vi "SeCrTs-RD AI Indexing.vi"(11 "AI Config":T1) -> ()   [LabVIEW 2022 SP3]
panel:
  out "Ai Index Element":i32[](array[numeric])
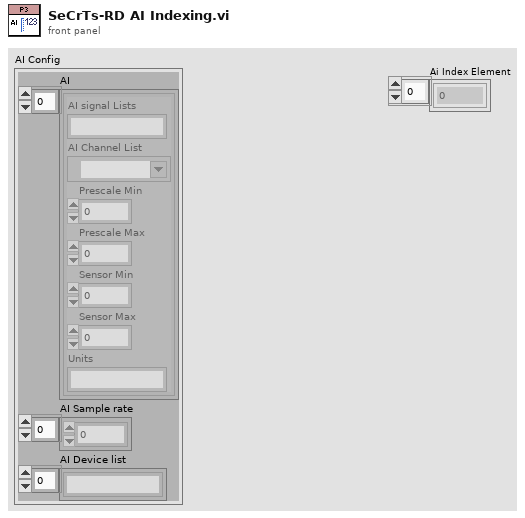
[diagram p1: front panel]
types:
  T1 = cluster{"AI":cluster{"AI signal Lists":string, "AI Channel List":tag, "Prescale Min":dbl, "Prescale Max":dbl, "Sensor Min":dbl, "Sensor Max":dbl, "Units":string}[], "AI Sample rate":i32[], "AI Device list ":string[]}
  T2 = cluster{"AI signal Lists":string, "AI Channel List":tag, "Prescale Min":dbl, "Prescale Max":dbl, "Sensor Min":dbl, "Sensor Max":dbl, "Units":string}[]
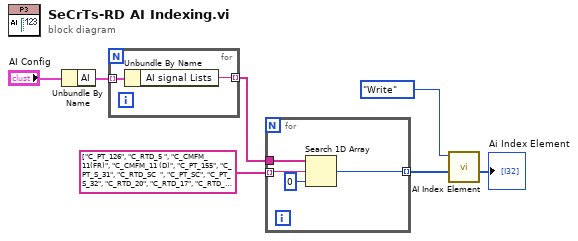
[diagram p0: block diagram]
diagram:
  n1 = Unbundle By Name("AI Config") -> ("AI"=w5:T2)
  n2 = for {
    tunnel: [w9] -> w7 mode=indexing
    tunnel: w5 -> [w8] mode=indexing
    n3 = Unbundle By Name(w8) -> ("AI signal Lists"=w9:string)
  }
  n4 = for {
    tunnel: w7 -> [w13]
    tunnel: string[] ["C_PT_126", "C_RTD_5 ", "C_CMFM_11(FR)", "C_CMFM_11 (D)", "C_PT_155", "C_PT_S_31", "C_RTD_SC  ", "C_PT_SC", "C_PT_S_32", "C_RTD_20", "C_RTD_17", "C_RTD_13a", "C_PT_13a", "C_PT_13c", "G_PT_51", "G_CMFM_53(D)", "G_CMFM_53 (FR)", "C_PT_55", "N_PT_1351", "F_RTD_31b ", "F_PT_ 31b", "E_PT_CC5", "E_PT_CC2", "E_PT_CC3", "E_PT_CC4", "F_PT_29c", "F_PT_29b", "I_TC", "E_TC_inj2", "I_MPT", "C_PT_13d", "C_PT_13b", "C_RTD_13b", "F_RTD_31a", "F_PT_31a", "E_TC_CC", "F_RTD_Regen1", "F_RTD_Regen2", "E_TC_ET", "F_PT_135", "F_PT_129a", "F_PT_129b", "F_PT_24", "F_CMFM_27(D)", "F_CMFM_27 (FR)", "F_PT_32", "F_PT_SC", "F_RTD_SC", "F_PT_31", "F_RTD_29", "F_PT_29 a ", "F_PT_49", "F_CMFM_43(FR)", "F_CMFM_43(D)", "C_PT_45"] -> [w12] mode=indexing
    tunnel: [w10] -> w2 mode=indexing
    n5 = Search 1D Array(1D array=w13, element=w12, start index (0)=0) -> (index of element=w10:i32)
  }
  n6 = call "AI Index Element.vi"("AI Index Element"=w2, "Write/Read"=enum16{"Write", "Read"}."Write") -> ("Ai Index Element"=→"Ai Index Element":i32[])  [unwired: 9 in]
